vi "Contour Line_Check Intersected Edges.vi"(6 "row? (F)":bool, 7 "Z":dbl[][](array[numeric]), 8 "height":dbl, 9 "edge in":T1, 10 "Y":dbl[][](array[numeric]), 11 "X":dbl[][](array[numeric])) -> (1 "edge out":T1, 2 "contour point":cluster{"x":dbl, "y":dbl}, 3 "intersected?":bool)   [LabVIEW 2020, in "NI_AAL_Geometry.lvlib"]
uses:
  <vilib>/Analysis/NI_AAL_Geometry.lvlib
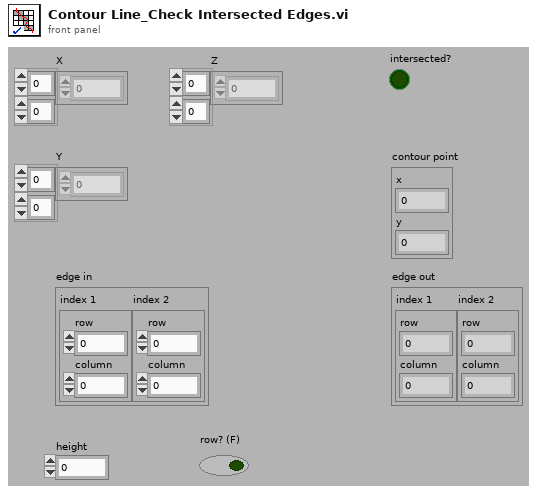
[diagram p1: front panel]
types:
  T1 = cluster{"index 1":cluster{"row":i32, "column":i32}, "index 2":cluster{"row":i32, "column":i32}}
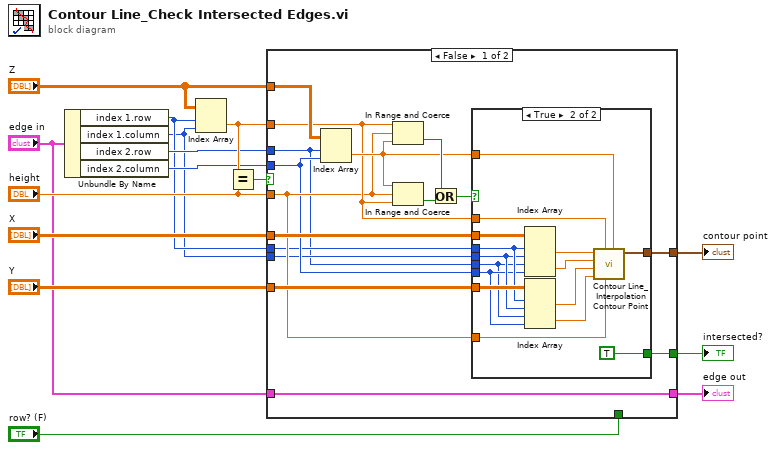
[diagram p0: block diagram]
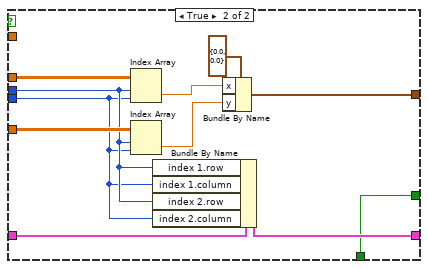
[diagram p3: hidden frame]
diagram:
  n1 = Unbundle By Name("edge in") -> ("index 1.row"=w6:i32, "index 1.column"=w5:i32, "index 2.row"=w11:i32, "index 2.column"=w10:i32)
  n2 = Index Array(array="Z", index (row)=w6, index (col)=w5) -> (element=w14:dbl)
  n3 = Equal?(x=w14, y="height") -> (x = y?=w15:bool)
  n4 = case shown="False" w15 {
    tunnel: "Z" -> [w31 _]
    tunnel: w14 -> [w26 _]
    tunnel: w11 -> [w18 _]
    tunnel: w10 -> [w21 _]
    tunnel: "height" -> [w23 _]
    tunnel: "X" -> [w25 w57]
    tunnel: "Y" -> [w24 w56]
    tunnel: [w22 w52] -> w7
    tunnel: w6 -> [w20 w50]
    tunnel: w5 -> [w19 w49]
    tunnel: [w17 w47] -> w4
    tunnel: "edge in" -> [w16 w51]
    tunnel: [w16 w48] -> w2
    tunnel: "row? (F)" -> [_ w47]
    frame False {
      n5 = Index Array(array=w31, index (row)=w18, index (col)=w21) -> (element=w27:dbl)
      n6 = In Range and Coerce(upper limit=w26, x=w23, lower limit=w27) -> (In Range?=w29:bool)  [unwired: 1 out]
      n7 = In Range and Coerce(upper limit=w27, x=w23, lower limit=w26) -> (In Range?=w30:bool)  [unwired: 1 out]
      n8 = Or(x=w29, y=w30) -> (x .or. y?=w28:bool)
      n9 = case shown="True" w28 {
        tunnel: w27 -> [_ w45]
        tunnel: w26 -> [_ w46]
        tunnel: w25 -> [_ w44]
        tunnel: w20 -> [_ w37]
        tunnel: w19 -> [_ w36]
        tunnel: w21 -> [_ w35]
        tunnel: w24 -> [_ w43]
        tunnel: w23 -> [_ w38]
        tunnel: [_ w34] -> w22
        tunnel: w18 -> [_ w33]
        tunnel: [_ TRUE] -> w17
        frame False {
        }
        frame True {
          n10 = Index Array(array=w44, index (row) #1=w37, index (col) #1=w36, index (row) #2=w33, index (col) #2=w35) -> (element #1=w42:dbl, element #2=w41:dbl)
          n11 = Index Array(array=w43, index (row) #1=w37, index (col) #1=w36, index (row) #2=w33, index (col) #2=w35) -> (element #1=w40:dbl, element #2=w39:dbl)
          n12 = call <vilib>:"Contour Line_Interpolation Contour Point.vi"("z 2"=w45, "height"=w38, "z 1"=w46, "y 2"=w39, "y 1"=w40, "x 2"=w41, "x 1"=w42) -> ("contour point"=w34:cluster{"x":dbl, "y":dbl})  [unwired: 4 out]
        }
      }
    }
    frame True {
      n13 = Index Array(array=w57, index (row)=w50, index (col)=w49) -> (element=w54:dbl)
      n14 = Index Array(array=w56, index (row)=w50, index (col)=w49) -> (element=w53:dbl)
      n15 = Bundle By Name(cluster=w51, "index 1.row"=w50, "index 1.column"=w49, "index 2.row"=w50, "index 2.column"=w49) -> (w48:T1)
      n16 = Bundle By Name(cluster=cluster{"x":dbl, "y":dbl} {"x"=0.0, "y"=0.0} ("contour point"), "x"=w54, "y"=w53) -> (w52:cluster{"x":dbl, "y":dbl})
    }
  }
  "contour point" <- w7
  "edge out" <- w2
  "intersected?" <- w4
